vi "Lunch and Learn Async.vi"() -> ()   [LabVIEW 2016]
panel:
  in  "State":enum16{"By Ref", "By Invoke Node"}(ring)
  out "error out":errorcluster
  in  "error in (no error)":errorcluster
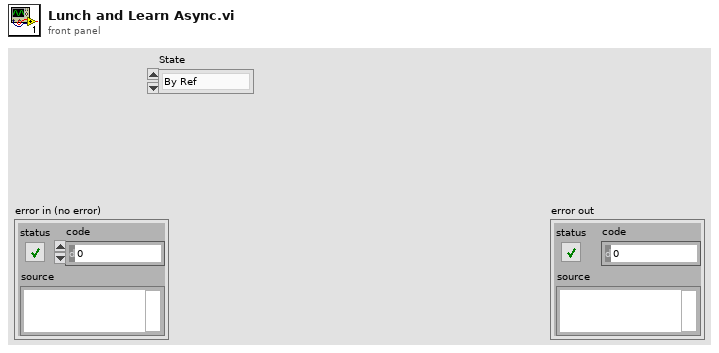
[diagram p1: front panel]
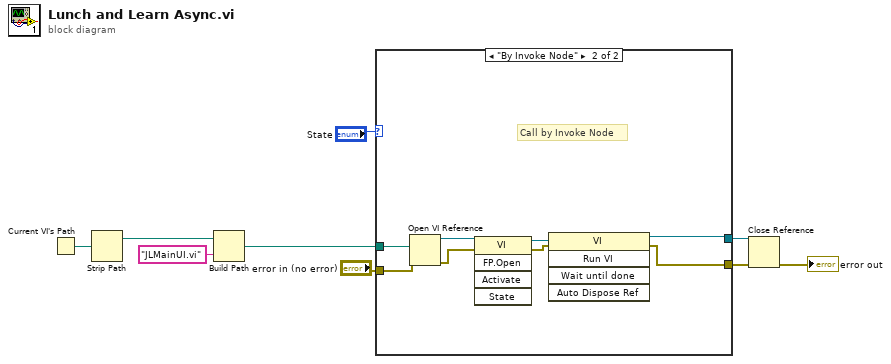
[diagram p0: block diagram]
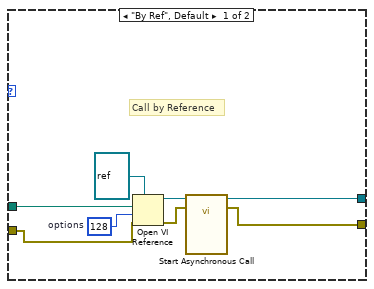
[diagram p2: hidden frame]
diagram:
  n1 = Current VI's Path() -> (path=w6:path)
  n2 = Strip Path(path=w6) -> (stripped path=w7:path)  [unwired: 1 out]
  n3 = Build Path(base path=w7, name or relative path="JLMainUI.vi") -> (appended path=w5:path)
  n4 = case shown="\"By Invoke Node\"" "State" {
    tunnel: "error in (no error)" -> [w13 w18]
    tunnel: w5 -> [w12 w25]
    tunnel: [w11 w22] -> w4
    tunnel: [w10 w21] -> w3
    frame "By Ref", Default {
      w17 = 128  # options
      # "Call by Reference"
      n5 = Open VI Reference(type specifier VI Refnum (for type only)=refnum<vi> refnum ("reference"), vi path=w12, options=w17, error in (no error)=w13) -> (vi reference=w15:refnum<vi>, error out=w16:errorcluster)  [unwired: 2 in]
      n6 = call-by-ref "Start Asynchronous Call"(reference=w15, error in=w16) -> (reference out=w11:refnum<vi>, error out=w10:errorcluster)  [unwired: 10 in, 2 out]
    }
    frame "By Invoke Node" {
      # "Call by Invoke Node"
      n7 = Open VI Reference(vi path=w25, error in (no error)=w18) -> (vi reference=w24:refnum<vi>, error out=w19:errorcluster)  [unwired: 4 in]
      n8 = invoke class="VI" method="FP.Open"(reference=w24, error in=w19) -> (reference out=w23:refnum<vi>, error out=w20:errorcluster)  [unwired: 3 in, 3 out]
      n9 = invoke class="VI" method="Run VI"(reference=w23, error in=w20) -> (reference out=w22:refnum<vi>, error out=w21:errorcluster)  [unwired: 3 in, 3 out]
    }
  }
  n10 = Close Reference(reference=w4, error in (no error)=w3) -> (error out=→"error out":errorcluster)
